vi "test Copy To Larger Destinationvi.vi"(8 "error in (no error)":errorcluster, 11 "TestCase in":refnum<class "Data Manipulation Tests.lvclass">) -> (0 "error out":errorcluster, 3 "TestCase out":refnum<class "Data Manipulation Tests.lvclass">)   [LabVIEW 2017, in "Pointer Tests.lvlib" / "Data Manipulation Tests.lvclass"]
uses:
  Data Manipulation Tests.lvclass
  Source/Classes/Pointer/Public/New/New (4B).vi
  Source/Classes/Pointer/Public/Write/Write (1D I32).vi
  Source/Classes/Pointer/Public/New/New (8B).vi
  Source/Classes/Pointer/Public/Read/Read (1D I32).vi
  <vilib>/addons/_JKI Toolkits/VI Tester/TestCase.llb/TestCase.lvclass
  Source/Classes/Pointer/Pointer.lvclass
  C:/Program Files (x86)/National Instruments/LabVIEW 2017/vi.lib/addons/_JKI Toolkits/VI Tester/TestCase.llb/TestCase.lvclass
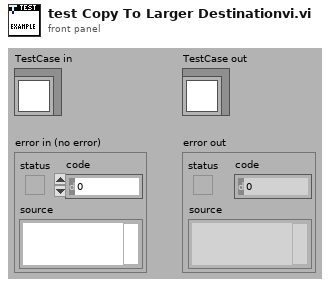
[diagram p1: front panel]
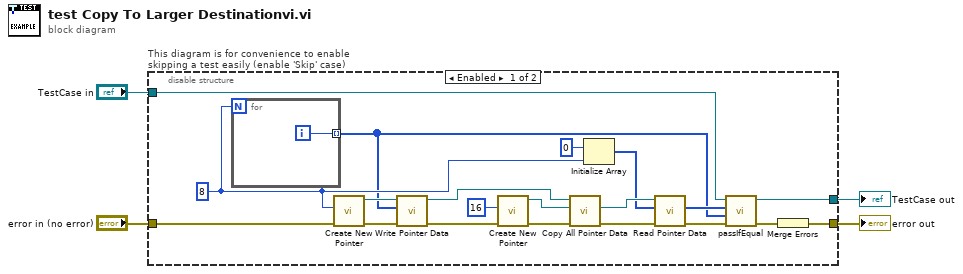
[diagram p0: block diagram]
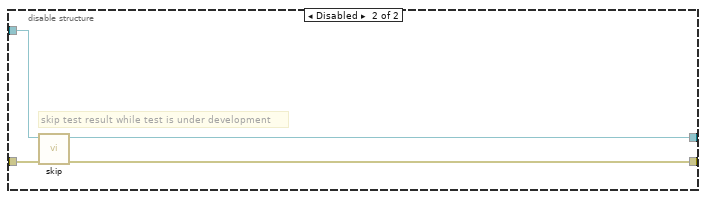
[diagram p2: hidden frame]
diagram:
  n1 = disable-structure "This diagram is for convenience to enable skipping a test easily (enable 'Skip' case)" shown="Enabled" {
    disable-tunnel: "TestCase in" -> [w13 w29]
    disable-tunnel: [w12 w27] -> w1
    disable-tunnel: [w18 w28] -> w3
    disable-tunnel: "error in (no error)" -> [w17 w26]
    frame Enabled {
      w10 = u64 8 ("count (1)")
      n2 = for {
        N: w10 -> [_]
        tunnel: [w25] -> w7 mode=indexing
        i -> [w25]
      }
      n3 = call-poly "Create New Pointer.vi"("error in (no error)"=w17, "count (1)"=w10) -> ("error out"=w21:errorcluster, "Pointer"=w24:refnum<class "Pointer.lvclass">)  [unwired: 8 in]
      n4 = call-poly "Write Pointer Data.vi"("error in (no error)"=w21, "buffer in"=w7, "Pointer in"=w24) -> ("error out"=w20:errorcluster, "Pointer out"=w23:refnum<class "Pointer.lvclass">)  [unwired: 5 in, 2 out]
      n5 = call-poly "Create New Pointer.vi"("error in (no error)"=w20, "count (1)"=u64 16) -> ("error out"=w19:errorcluster, "Pointer"=w22:refnum<class "Pointer.lvclass">)  [unwired: 8 in]
      n6 = call "Copy All Pointer Data.vi"("error in (no error)"=w19, "dst Pointer in"=w22, "src Pointer in"=w23) -> ("error out"=w6:errorcluster, "dst Pointer out"=w15:refnum<class "Pointer.lvclass">)  [unwired: 6 in, 1 out]
      n7 = Initialize Array(0 ("element"), w10) -> (w8:i32[])
      n8 = call-poly "Read Pointer Data.vi"("error in (no error)"=w6, "buffer in"=w8, "Pointer in"=w15) -> ("error out"=w5:errorcluster, "buffer out"=w11:i32[])  [unwired: 5 in, 2 out]
      n9 = call-dynamic "passIfEqual.vi"("error in (no error)"=w5, "y"=w7, "x"=w11, "TestCase in"=w13) -> ("error out"=w14:errorcluster, "TestCase out"=w12:refnum<class "Data Manipulation Tests.lvclass">)  [unwired: 6 in]
      n10 = Merge Errors(w14) -> (w18:errorcluster)
    }
    frame Disabled {
      # "skip test result while test is under development"
      n11 = call <vilib>:"skip.vi"("error in (no error)"=w26, "TestCase in"=w29) -> ("error out"=w28:errorcluster, "TestCase out"=w27:refnum<class "Data Manipulation Tests.lvclass">)  [unwired: 8 in]
    }
  }
  "error out" <- w3
  "TestCase out" <- w1
